vi "solar_cfg Write (Section).vi"(0 "Config Refnum in":refnum<data-value>, 1 "Section":string, 2 "Comment (New section only)":string, 11 "error in (no error)":errorcluster) -> (4 "Config Refnum out":refnum<data-value>, 10 "Found?":bool, 15 "error out":errorcluster)   [LabVIEW 2018]
doc: "Create a configure file section '[SECTION]'. The comment is only written if the section does not exist."
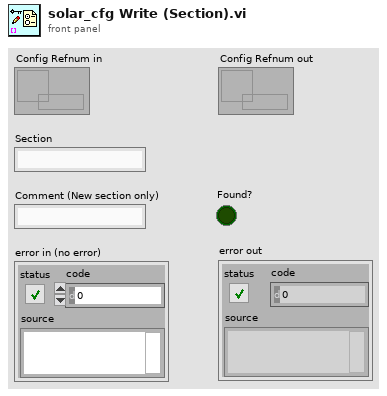
[diagram p1: front panel]
types:
  T1 = cluster{"Dirty":bool, "Semaphore":refnum<queue>, "Sections":cluster{"Section":string, "kvc":string[][]}[], "Path":path}
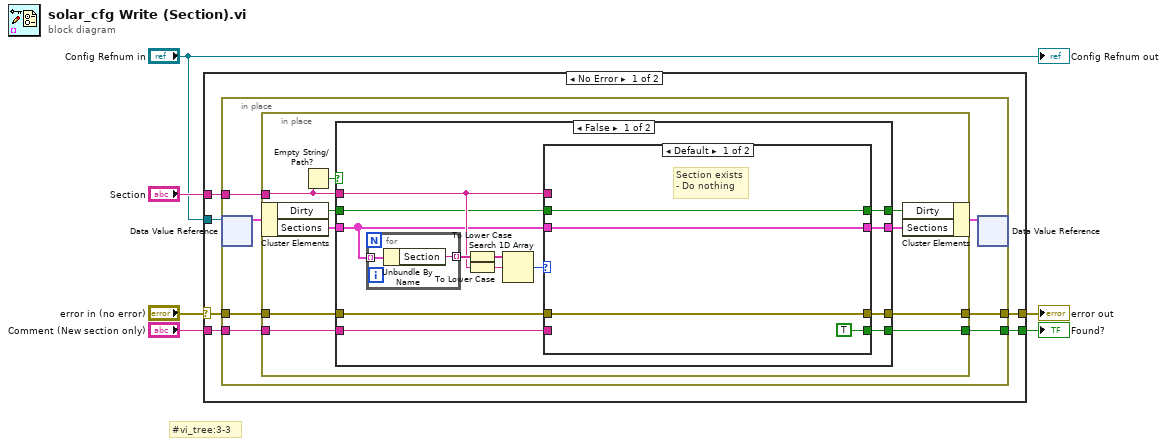
[diagram p0: block diagram]
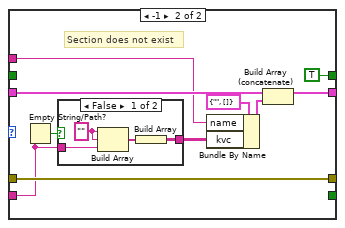
[diagram p2: hidden frame]
diagram:
  # "#vi_tree:3-3"
  n1 = case shown="No Error" "error in (no error)" {
    selector: "error in (no error)" -> [w12 w66]
    tunnel: [w11 w66] -> w2
    tunnel: "Config Refnum in" -> [w10 _]
    tunnel: [w9 _] -> w1
    tunnel: "Comment (New section only)" -> [w8 _]
    tunnel: "Section" -> [w7 _]
    frame No Error {
      n2 = in-place {
        in-place-border: w12 -> [w19]
        in-place-border: [w18] -> w11
        in-place-border: w8 -> [w17]
        in-place-border: w7 -> [w16]
        in-place-border: [w13] -> w9
        n3 = in-place-dvr #1(w10) -> (w15:T1)  [unwired: 1 out]
        n4 = in-place {
          in-place-border: w19 -> [w24]
          in-place-border: [w29] -> w18
          in-place-border: w17 -> [w28]
          in-place-border: w16 -> [w21]
          in-place-border: [w25] -> w13
          n5 = in-place-cluster #2(w15) -> ("Dirty"=w22:bool, "Sections"=w23:cluster{"Section":string, "kvc":string[][]}[])
          n6 = Empty String/Path?(string/path=w21) -> (empty?=w20:bool)
          n7 = case shown="False" w20 {
            tunnel: [w42 w63] -> w29
            tunnel: w28 -> [w41 _]
            tunnel: [w40 w65] -> w27
            tunnel: [w39 w64] -> w26
            tunnel: [w38 _] -> w25
            tunnel: w24 -> [w37 w63]
            tunnel: w21 -> [w33 _]
            tunnel: w23 -> [w32 w65]
            tunnel: w22 -> [w30 w64]
            frame False {
              n8 = for {
                tunnel: w32 -> [w62] mode=indexing
                tunnel: [w61] -> w36 mode=indexing
                n9 = Unbundle By Name(w62) -> ("Section"=w61:string)
              }
              n10 = To Lower Case(string=w36) -> (all lower case string=w35:string[])
              n11 = To Lower Case(string=w33) -> (all lower case string=w34:string)
              n12 = Search 1D Array(1D array=w35, element=w34) -> (index of element=w31:i32)  [unwired: 1 in]
              n13 = case shown="Default" w31 {
                tunnel: [w44 w49] -> w42
                tunnel: w41 -> [_ w48]
                tunnel: [w46 w51] -> w40
                tunnel: [w45 TRUE ("Dirty")] -> w39
                tunnel: [TRUE ("Found?") _] -> w38
                tunnel: w37 -> [w44 w49]
                tunnel: w33 -> [_ w52]
                tunnel: w32 -> [w46 w53]
                tunnel: w30 -> [w45 _]
                frame Default {
                  # "Section exists\n- Do nothing"
                }
                frame -1 {
                  # "Section does not exist"
                  n14 = Empty String/Path?(string/path=w48) -> (empty?=w47:bool)
                  n15 = case shown="False" w47 {
                    tunnel: [w59 _] -> w54
                    tunnel: w48 -> [w58 _]
                    frame False {
                      w57 = "" ("element")
                      n16 = Build Array(w57, w57, w58) -> (w60:string[])
                      n17 = Build Array(w60) -> (w59:string[][])
                    }
                    frame True {
                    }
                  }
                  n18 = Bundle By Name(cluster=cluster{"name":string, "kvc":string[][]} {"name"="", "kvc"=[]} ("Section"), "name"=w52, "kvc"=w54) -> (w55:cluster{"name":string, "kvc":string[][]})
                  n19 = Build Array (concatenate)(w53, w55) -> (w51:cluster{"name":string, "kvc":string[][]}[])
                }
              }
            }
            frame True {
            }
          }
          n20 = in-place-cluster #2("Dirty"=w26, "Sections"=w27) -> (w14:T1)
        }
        n21 = in-place-dvr #1(w14) -> ()  [unwired: 2 out]
      }
    }
    frame Error {
    }
  }
  "error out" <- w2
  "Found?" <- w1
  "Config Refnum out" <- "Config Refnum in"
